vi "TX.vi"(5 "timeout in ms (-1)":i32, 7 "TCP Queue":refnum<queue>, 8 "error in (no error)":errorcluster, 9 "PDU_req":T1={"Function Code"=1, "Data"=[], "RTU_DataBytes"=0}, 10 "Transaction LUT in":refnum<data-value>, 11 "ADU in":refnum<class "MB_ADU_TCP.lvclass">) -> (0 "error out":errorcluster, 1 "Transaction Notifier":refnum<notifier>, 2 "Transaction LUT out":refnum<data-value>, 3 "ADU out":refnum<class "MB_ADU_TCP.lvclass">)   [LabVIEW 2016, in "MB Master.lvlib" / "MB_Master_TCP.lvclass"]
uses:
  MB_Master_TCP.lvclass
  MB_ADU_TCP/MB_ADU_TCP.lvclass
  MB_PDU/MB_PDU_Cluster.ctl
  MB_ADU_TCP/MB_ADU_TCP.lvclass/MB_ADU_TCP.ctl
  MB_ADU_TCP/Write Transaction ID.vi
  MB Master.lvlib
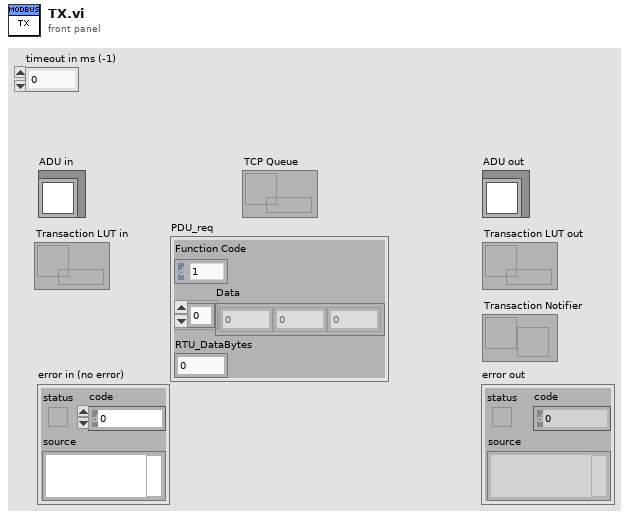
[diagram p1: front panel]
types:
  T1 = typedef "MB Master.lvlib/MB_PDU_Cluster.ctl" = cluster{"Function Code":u8, "Data":u8[], "RTU_DataBytes":i32}
  T2 = cluster{"TX Data":string, "notifier out":refnum<notifier>}
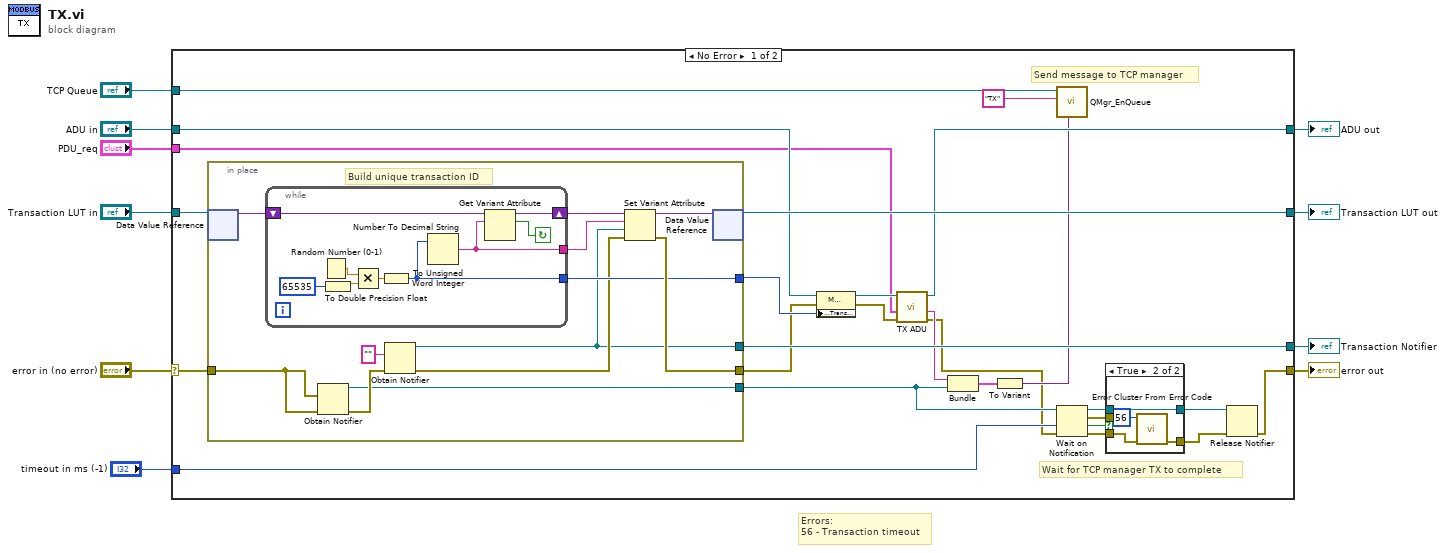
[diagram p0: block diagram]
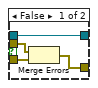
[diagram p2: hidden frame]
diagram:
  # "Errors:\n56 - Transaction timeout"
  n1 = case shown="No Error" "error in (no error)" {
    selector: "error in (no error)" -> [w36 w68]
    tunnel: [w12 w68] -> w9
    tunnel: "Transaction LUT in" -> [w35 w67]
    tunnel: [w34 w67] -> w7
    tunnel: [w33 _] -> w6
    tunnel: "ADU in" -> [w30 w66]
    tunnel: "TCP Queue" -> [w25 _]
    tunnel: [w27 w66] -> w3
    tunnel: "PDU_req" -> [w26 _]
    tunnel: "timeout in ms (-1)" -> [w19 _]
    frame No Error {
      # "Wait for TCP manager TX to complete"
      # "Send message to TCP manager"
      n2 = in-place {
        in-place-border: w36 -> [w47]
        in-place-border: [w56] -> w28
        in-place-border: [w54] -> w29
        in-place-border: [w52] -> w33
        in-place-border: [w45] -> w20
        # "Build unique transaction ID"
        n3 = in-place-dvr #1(w35) -> (w50:variant)  [unwired: 1 out]
        n4 = while {
          tunnel: [w59] -> w51
          tunnel: [w61] -> w54
          shift-right: [w58] -> w49
          shift-left: w50 -> [w60]
          stop <- w57 continue-if-true
          n5 = Random Number (0-1)() -> (number: 0 to 1=w65:dbl)
          n6 = To Double Precision Float(number=u16 65535) -> (double precision float=w63:dbl)
          n7 = Multiply(x=w65, y=w63) -> (x*y=w62:dbl)
          n8 = To Unsigned Word Integer(number=w62) -> (unsigned 16bit integer=w61:u16)
          n9 = Number To Decimal String(number=w61) -> (decimal integer string=w59:string)  [unwired: 1 in]
          n10 = Get Variant Attribute(Variant=w60, name=w59) -> (duplicate Variant=w58:variant, found=w57:bool)  [unwired: 2 in, 2 out]
        }
        n11 = Obtain Notifier(notification data type=w47, error in (no error)=w47) -> (notifier out=w45:refnum<notifier>, error out=w46:errorcluster)  [unwired: 2 in, 1 out]
        n12 = Obtain Notifier(notification data type="", error in (no error)=w46) -> (notifier out=w52:refnum<notifier>, error out=w53:errorcluster)  [unwired: 2 in, 1 out]
        n13 = Set Variant Attribute(Variant=w49, name=w51, value=w52, error in=w53) -> (Variant out=w55:variant, error out=w56:errorcluster)  [unwired: 1 out]
        n14 = in-place-dvr #1(w55) -> (w34:refnum<data-value>)  [unwired: 1 out]
      }
      n15 = property class="MB_ADU_TCP"(reference=w30, error in=w28, "Properties:Transaction ID"=w29) -> (reference out=w31:refnum<class "MB_ADU_TCP.lvclass">, error out=w32:errorcluster)
      n16 = call "TX ADU.vi"("error in (no error)"=w32, "PDU_req in"=w26, "MB_ADU_TCP in"=w31) -> ("error out"=w15:errorcluster, "TX Data"=w22:string, "MB_ADU_TCP out"=w27:refnum<class "MB_ADU_TCP.lvclass">)  [unwired: 6 in]
      n17 = Bundle("TX Data"=w22, "notifier out"=w20) -> (w21:T2)  [unwired: 1 in]
      n18 = To Variant(anything=w21) -> (Variant=w23:variant)
      n19 = call "QMgr_EnQueue.vi"("Data"=w23, "Command"="TX", "queue in"=w25) -> ()  [unwired: 8 in, 1 out]
      n20 = Wait on Notification(notifier=w20, timeout in ms (-1)=w19, error in (no error)=w15) -> (notifier out=w14:refnum<notifier>, notification=w17:errorcluster, timed out?=w16:bool, error out=w18:errorcluster)  [unwired: 1 in]
      n21 = case shown="True" w16 {
        tunnel: w18 -> [w40 w43]
        tunnel: w17 -> [w39 _]
        tunnel: [w38 w42] -> w11
        tunnel: w14 -> [w37 w41]
        tunnel: [w37 w41] -> w13
        frame False {
          n22 = Merge Errors(w39, w40) -> (w38:errorcluster)
        }
        frame True {
          n23 = call <vilib>:"Error Cluster From Error Code.vi"("error in (no error)"=w43, "error code (0)"=56) -> ("error out"=w42:errorcluster)  [unwired: 7 in]
        }
      }
      n24 = Release Notifier(notifier=w13, error in (no error)=w11) -> (error out=w12:errorcluster)  [unwired: 1 in, 2 out]
    }
    frame Error {
    }
  }
  "error out" <- w9
  "Transaction LUT out" <- w7
  "Transaction Notifier" <- w6
  "ADU out" <- w3
